vi "cmd_set_ao_range.vi"(8 "error in (no error)":errorcluster, 11 "JSON":string) -> (0 "error out":errorcluster)   [LabVIEW 2021]
doc: "Set the maximum and minimum analogue output values. \n\n :param low: Specifies the lower limit of the output (8ch)\n :param high: Specifies the higher limit of the output (8ch)"
uses:
  core/host_global_vars.vi
  <vilib>/Utility/error.llb/Error Cluster From Error Code.vi
  <vilib>/rvi/errors/niLvFpgaAdjustHostInterfaceError.vi
  <vilib>/rvi/interface/nirviReadWriteControl/nirviReadWriteControl.xnode
  fpga/fpga_dtype_sgl_8ch.ctl
  FPGA Bitfiles/openlabspm_FPGATarget_fpgamain_eo-gUZR5D1g.lvbitx
  fpga/fpga_main.vi
  NiFpgaLv.dll
panel:
  in  "args":cluster{"low":sgl[], "high":sgl[]}
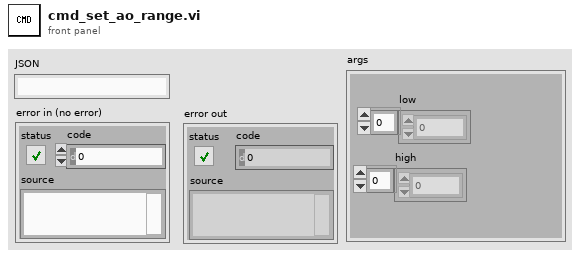
[diagram p1: front panel]
types:
  T1 = cluster{"low[0]":sgl, "low[1]":sgl, "low[2]":sgl, "low[3]":sgl, "low[4]":sgl, "low[5]":sgl, "low[6]":sgl, "low[7]":sgl}
  T2 = cluster{"high[0]":sgl, "high[1]":sgl, "high[2]":sgl, "high[3]":sgl, "high[4]":sgl, "high[5]":sgl, "high[6]":sgl, "high[7]":sgl}
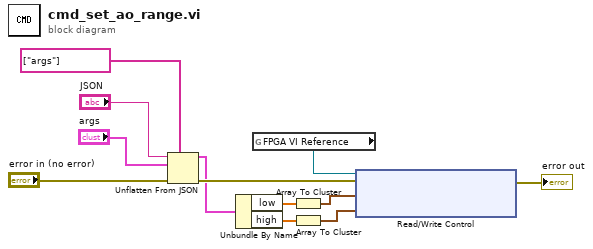
[diagram p0: block diagram]
diagram:
  n1 = Unflatten From JSON(path=string[] ["args"], JSON string="JSON", type and defaults="args", error in (no error)="error in (no error)") -> (value=w5:cluster{"low":sgl[], "high":sgl[]}, error out=w7:errorcluster)  [unwired: 3 in]
  n2 = Unbundle By Name(w5) -> ("low"=w4:sgl[], "high"=w3:sgl[])
  n3 = global read "host_global_vars.vi" "FPGA VI Reference"() -> (w8:refnum<k20>)
  n4 = Array To Cluster(array=w4) -> (cluster=w2:T1)
  n5 = Array To Cluster(array=w3) -> (cluster=w1:T2)
  n6 = xnode "Read/Write Control"("FPGA VI Reference In"=w8, "error in"=w7, "limit (low, 10 V)"=w2, "limit (high, 10 V)"=w1) -> ("error out"=→"error out":errorcluster)  [unwired: 1 out]
